vi "pixStatusConvert.vi"(7 "format string":string, 10 "error in":errorcluster, 11 "Hex Input String":string) -> (2 "error out":errorcluster, 3 "Pix No.":u16, 5 "En/Dis?":bool)   [LabVIEW 2018]
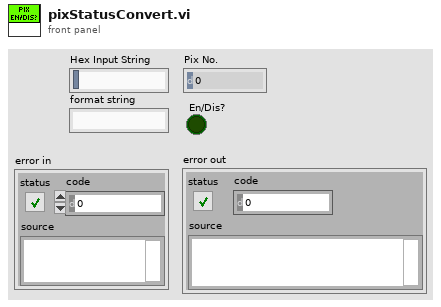
[diagram p1: front panel]
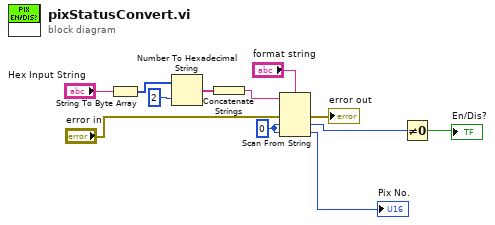
[diagram p0: block diagram]
diagram:
  w8 = u16 0 ("default value 1")
  n1 = String To Byte Array(string="Hex Input String") -> (unsigned byte array=w9:u8[])
  n2 = Number To Hexadecimal String(1:i16 2 ("Breite (-)"), 2:w9) -> (0:w11:string[])
  n3 = Concatenate Strings(w11) -> (w12:string)
  n4 = Scan From String(format string="format string", input string=w12, error in="error in", default 1=w8, default 2=w8) -> (error out=→"error out":errorcluster, output 1=w2:u16, output 2=→"Pix No.":u16)  [unwired: 1 in, 2 out]
  n5 = Not Equal To 0?(x=w2) -> (x != 0?=→"En/Dis?":bool)
